vi "Array Of Numbers.vi"(0 "Array 3":sgl[](array[numeric])=[337.0, 338.0, 339.0], 1 "Array 2":dbl[](array[numeric])=[224.0, 225.0, 226.0], 2 "Array":ext[](array[numeric])=[111.0, 112.0, 113.0], 3 "Array 11":cdb[](array[numeric])=[334.0+44.0i, 335.0+44.0i, 336.0+44.0i], 5 "Array 4":i32[](array[numeric])=[441, 442, 443], 6 "Array 15":fxp<+/-,64,32>[](array[numeric]), 7 "Array 5":i16[](array[numeric])=[554, 555, 556], 8 "Array 14":u64[](array[numeric])=[7788, 8855, 9955], 9 "Array 6":i8[](array[numeric])=[127, 127, 127], 10 "Array 13":i64[](array[numeric])=[5577, 5588, 5599], 11 "Array 7":u32[](array[numeric])=[771, 772, 773], 12 "Array 8":u16[](array[numeric])=[884, 885, 886], 13 "Array 9":u8[](array[numeric])=[255, 255, 255], 14 "Array 10":cxt[](array[numeric])=[111.0+22.0i, 112.0+22.0i, 113.0+22.0i], 15 "Array 12":csg[](array[numeric])=[557.0+66.0i, 558.0+66.0i, 559.0+66.0i]) -> ()   [LabVIEW 2009]
panel:
  in  "stop":bool
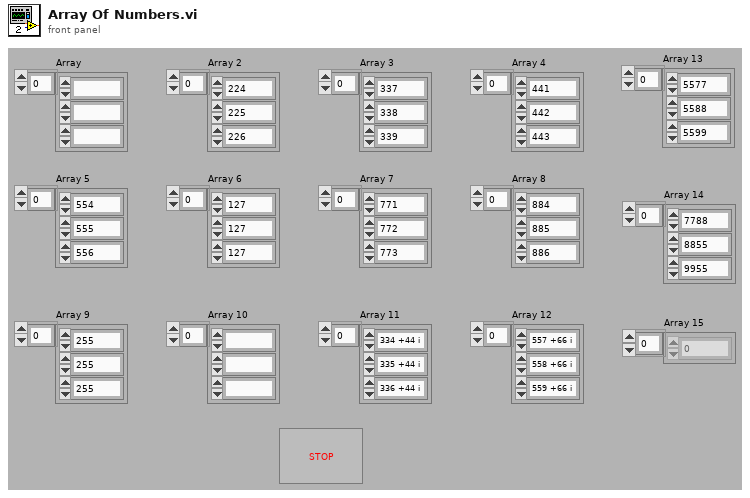
[diagram p1: front panel]
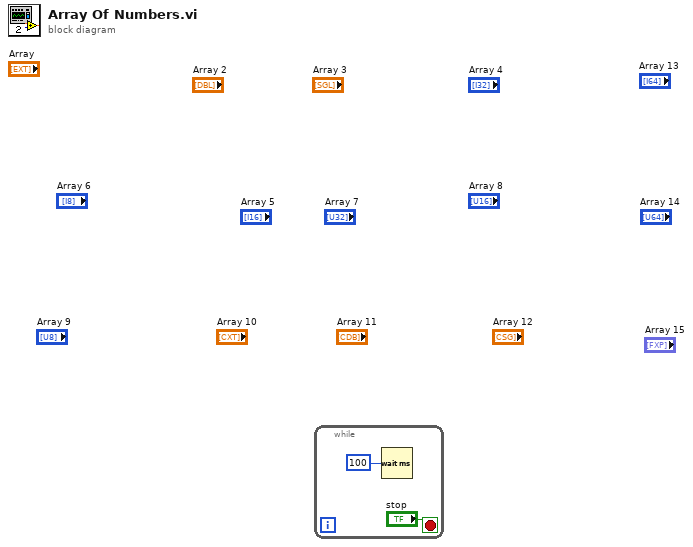
[diagram p0: block diagram]
diagram:
  n1 = while {
    stop <- "stop" stop-if-true
    n2 = Wait (ms)(milliseconds to wait=u32 100) -> ()  [unwired: 1 out]
  }
